vi "Lev-Mar xx with 2D encoded Gaussian.vi"(0 "fit type":u16, 5 "Standard Deviation":dbl[](array[numeric]) format="%.2f", 6 "code":dbl format="%.2f", 7 "error":i32, 8 "Coefficients":dbl[](array[numeric]) format="%.2f", 9 "Y":dbl[](array[numeric]) format="%.2f", 10 "X":dbl[](array[numeric]) format="%.2f") -> (4 "chiSqr":dbl format="%.2f")   [LabVIEW 2011]
doc: "This subprogram is derived from a subprogram contained in the National Instruments LabView advanced analysis library. The original subprogram is copyright National Instruments."
panel:
  # "Lev-Mar\nXX"
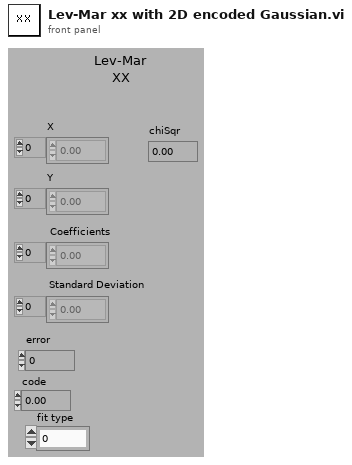
[diagram p1: front panel]
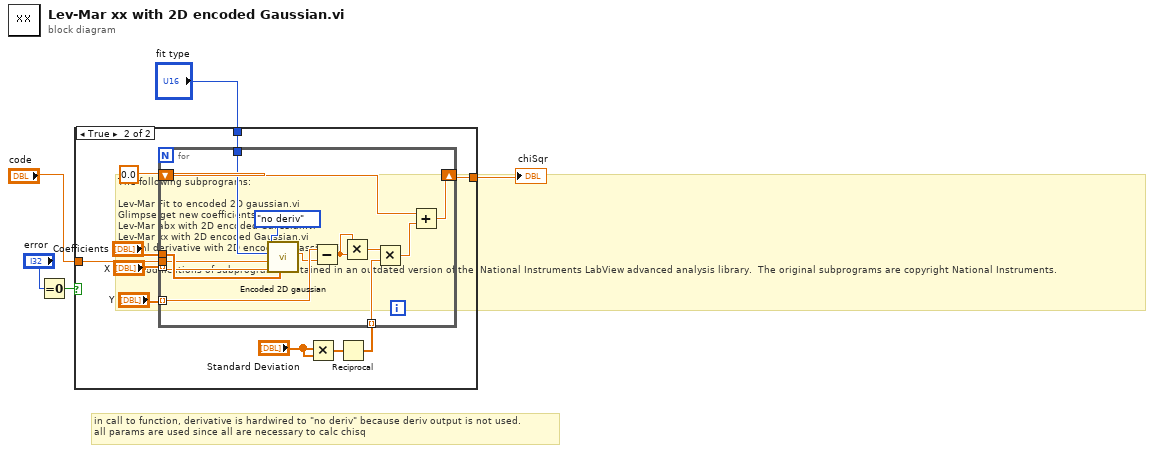
[diagram p0: block diagram]
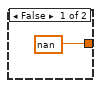
[diagram p2: hidden frame]
diagram:
  # "The following subprograms:\n\nLev-Mar Fit to encoded 2D gaussian.vi\nGlimpse get new coefficients.vi\nLev-Mar abx with 2D encoded Gaussian.vi\nLev-Mar xx with 2D encoded Gaussian.vi\npartial derivative with 2D encoded guassian.vi\n\nare modifications of subprograms contained in an outdated version of the  National Instruments LabView advanced analysis library.  The original subprograms are copyright National Instruments."
  # "in call to function, derivative is hardwired to \"no deriv\" because deriv output is not used.\nall params are used since all are necessary to calc chisq"
  n1 = Equal To 0?(x="error") -> (x = 0?=w4:bool)
  n2 = case shown="True" w4 {
    tunnel: [nan w15] -> w3
    tunnel: "code" -> [_ w8]
    tunnel: "fit type" -> [_ w7]
    frame False {
    }
    frame True {
      n3 = Multiply(x="Standard Deviation", y="Standard Deviation") -> (x*y=w10:dbl[])
      n4 = Reciprocal(x=w10) -> (1/x=w9:dbl[])
      n5 = for {
        shift-right: [w28] -> w15
        shift-left: 0.0 -> [w29]
        tunnel: "Y" -> [w27] mode=indexing
        tunnel: "Coefficients" -> [w25]
        tunnel: "X" -> [w24] mode=indexing
        tunnel: w9 -> [w19] mode=indexing
        tunnel: w8 -> [w18]
        tunnel: w7 -> [w17]
        n6 = call "Encoded 2D gaussian.vi"("Coefficients"=w25, "X"=w24, "code"=w18, "fit type"=w17, "Flag"=enum16{"no deriv", "deriv"}."no deriv") -> ("Y"=w23:dbl)  [unwired: 4 out]
        n7 = Subtract(x=w27, y=w23) -> (x-y=w26:dbl)
        n8 = Multiply(x=w26, y=w26) -> (x*y=w20:dbl)
        n9 = Multiply(x=w20, y=w19) -> (x*y=w21:dbl)
        n10 = Add(x=w29, y=w21) -> (x+y=w28:dbl)
      }
    }
  }
  "chiSqr" <- w3
